vi "RunMe (Test Launcher).vi"() -> ()   [LabVIEW 2013, in "Test Runner.AllAsserts.lvclass"]
uses:
  Test Runner.AllAsserts.lvclass
  classes/Test Runner/Test Runner.lvclass
panel:
  out "error out":errorcluster
  # "RUN ME.\n\nThis VI is an example of a Test Suite created as a Test Runner extension"
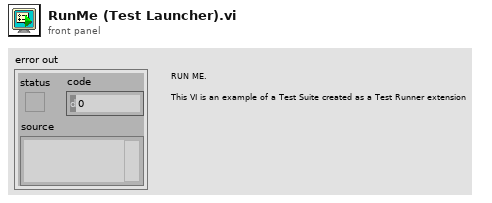
[diagram p1: front panel]
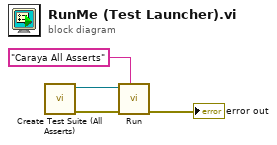
[diagram p0: block diagram]
diagram:
  n1 = call "Create Test Suite (All Asserts).vi"() -> ("error out"=w3:errorcluster, "Test Runner.AllAsserts in"=w4:refnum<class "Test Runner.AllAsserts.lvclass">)  [unwired: 10 in]
  n2 = call "Run.vi"("Name"="Caraya All Asserts", "error in (no error)"=w3, "Test Runner in"=w4) -> ("error out"=→"error out":errorcluster)  [unwired: 7 in, 1 out]
